vi "create_batchfile.vi"(0 "appended path":path, 1 "String 8":string, 2 "alternate path":path, 3 "String 6":string, 4 "String 4":string, 5 "String":string, 6 "String 5":string, 7 "Save in second location?":bool, 9 "String 2":string, 11 "String 3":string, 13 "String 9":string, 14 "String 10":string, 15 "String 7":string) -> ()   [LabVIEW 2013]
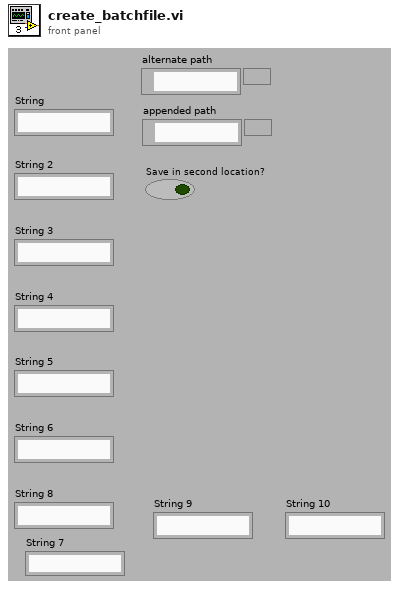
[diagram p1: front panel]
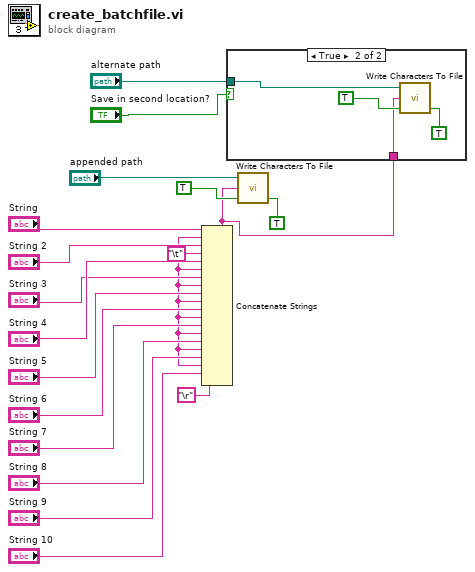
[diagram p0: block diagram]
diagram:
  w6 = "\t"
  n1 = Concatenate Strings("String", w6, "String 2", w6, "String 4", w6, "String 3", w6, "String 5", w6, "String 6", w6, "String 7", w6, "String 8", w6, "String 9", w6, "String 10", "\r") -> (w1:string)
  n2 = case shown="True" "Save in second location?" {
    tunnel: "alternate path" -> [_ w20]
    tunnel: w1 -> [_ w19]
    frame False {
    }
    frame True {
      n3 = call <vilib>:"Write Characters To File.vi"("convert eol? (no:F)"=TRUE, "append to file? (new file:F)"=TRUE, "character string"=w19, "file path (dialog if empty)"=w20) -> ()  [unwired: 1 in, 1 out]
    }
  }
  n4 = call <vilib>:"Write Characters To File.vi"("convert eol? (no:F)"=TRUE, "append to file? (new file:F)"=TRUE, "character string"=w1, "file path (dialog if empty)"="appended path") -> ()  [unwired: 1 in, 1 out]
